vi "test_Add Command_Check Existing Command Parameters Are Overwritten.vi"(8 "error in (no error)":errorcluster, 11 "TestCase in":refnum<class "Instrument Addon Scripting API Messages Unit Tests.lvclass">) -> (0 "error out":errorcluster, 3 "TestCase out":refnum<class "Instrument Addon Scripting API Messages Unit Tests.lvclass">)   [LabVIEW 2018, in "Instrument Addon Scripting API Messages Unit Tests.lvclass"]
uses:
  Instrument Addon Scripting API Messages Unit Tests.lvclass
  APIs/Scripting API/TypeDefs/Command Settings.ctl
  <vilib>/NI Veristand/Custom Device API/Custom Device Item Ref.ctl
  APIs/Scripting API/TypeDefs/Padding.ctl
  Addon/Addon Shared/Types/FG Control.ctl
  Addon/Addon Shared/Types/Command Parameters.ctl
  Addon/Addon Shared/Types/Linked Channel Cluster.ctl
  Instrument Addon Scripting API Messages Unit Tests.lvclass/Instrument Addon Scripting API Messages Unit Tests.ctl
  Addon/Addon Shared/SubVIs/Constants.vi
  <vilib>/NI/NI VeriStand Advanced SysDef API/_SubVIs/SysDef.Search.GUID.vi
  <vilib>/NI Veristand/Custom Device API/NI VeriStand - Get Item Property.vi
  <vilib>/NI Veristand/Custom Device API/Get Item Property (String).vi
  <vilib>/NI Veristand/Custom Device API/Get Item Property (String Array).vi
  <vilib>/NI Veristand/Custom Device API/Get Item Property (Boolean).vi
  <vilib>/NI Veristand/Custom Device API/Get Item Property (U32).vi
  <vilib>/NI Veristand/Custom Device API/NI VeriStand - Set Item Property.vi
  <vilib>/NI Veristand/Custom Device API/Set Item Property (String).vi
  <vilib>/NI Veristand/Custom Device API/Set Item Property (String Array).vi
  <vilib>/NI Veristand/Custom Device API/Set Item Property (Boolean).vi
  <vilib>/NI Veristand/Custom Device API/Set Item Property (U32).vi
  <vilib>/addons/_JKI Toolkits/VI Tester/TestCase.llb/TestCase.lvclass
  Instrument Addon Scripting API Test Assets/Instrument Addon Scripting API Test Assets.lvclass
  Addon/Addon Shared/Instrument Addon Shared.lvlib
  <vilib>/NI/NI VeriStand Advanced SysDef API/SysDef API/Advanced System Definition.lvlib
  <vilib>/NI Veristand/Custom Device API/Custom Device API.lvlib
  APIs/Scripting API/Instrument Addon Scripting API.lvlib
  C:/Program Files (x86)/National Instruments/LabVIEW 2018/vi.lib/addons/_JKI Toolkits/VI Tester/TestCase.llb/TestCase.lvclass
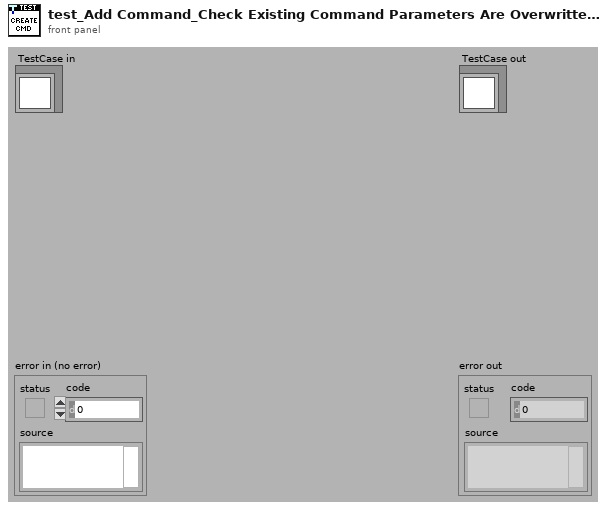
[diagram p1: front panel]
types:
  T1 = typedef "Instrument Addon Shared.lvlib/FG Control.ctl" = enum16{"Get", "Set"}
  T2 = typedef "Instrument Addon Scripting API.lvlib/Command Settings.ctl" = cluster{"Command Format":string, "Linked Channels":cluster{"Variable Name":string, "Channel Ref in":T3}[], "Use Padding?":bool, "Padding":T4}
  T3 = typedef "Custom Device API.lvlib/Custom Device Item Ref.ctl" = u64
  T4 = typedef "Instrument Addon Scripting API.lvlib/Padding.ctl" = cluster{"Pad Value":u8, "Length":u32}
  T5 = typedef "Instrument Addon Shared.lvlib/Command Parameters.ctl" = cluster{"Command":string, "Linked Channels":T6[], "Pad":bool, "Length":u32, "Pad Value":u8}
  T6 = typedef "Instrument Addon Shared.lvlib/Linked Channel Cluster.ctl" = cluster{"Variable Name":string, "GUID":string}
  T7 = typedef "Instrument Addon Scripting API.lvlib/Linked Channel.ctl" = cluster{"Variable Name":string, "Channel Refnum":T3}
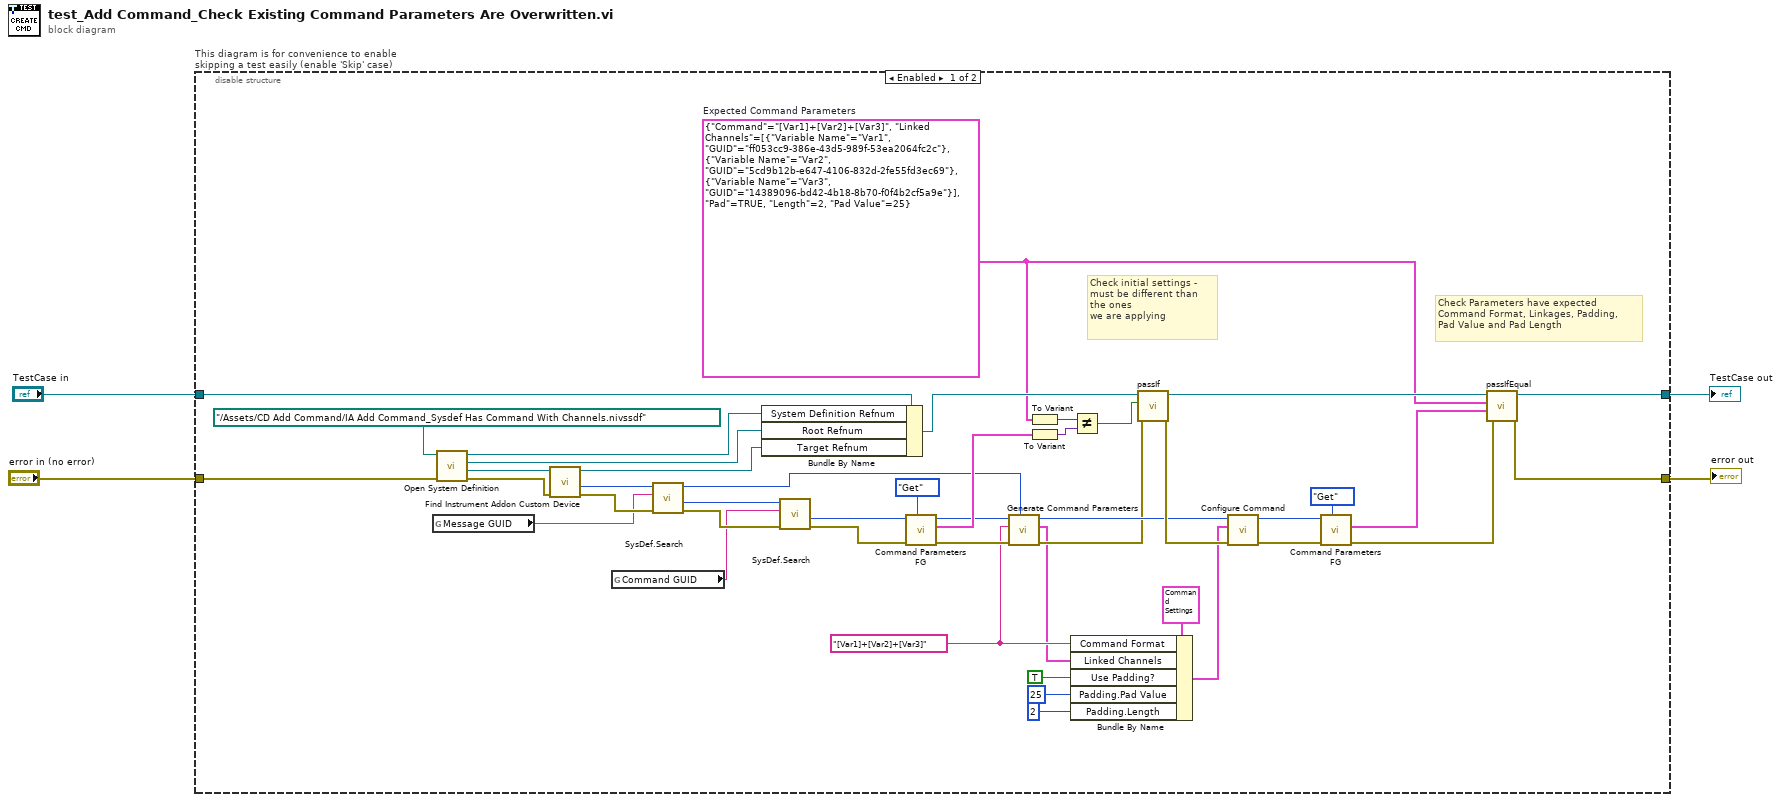
[diagram p0: block diagram]
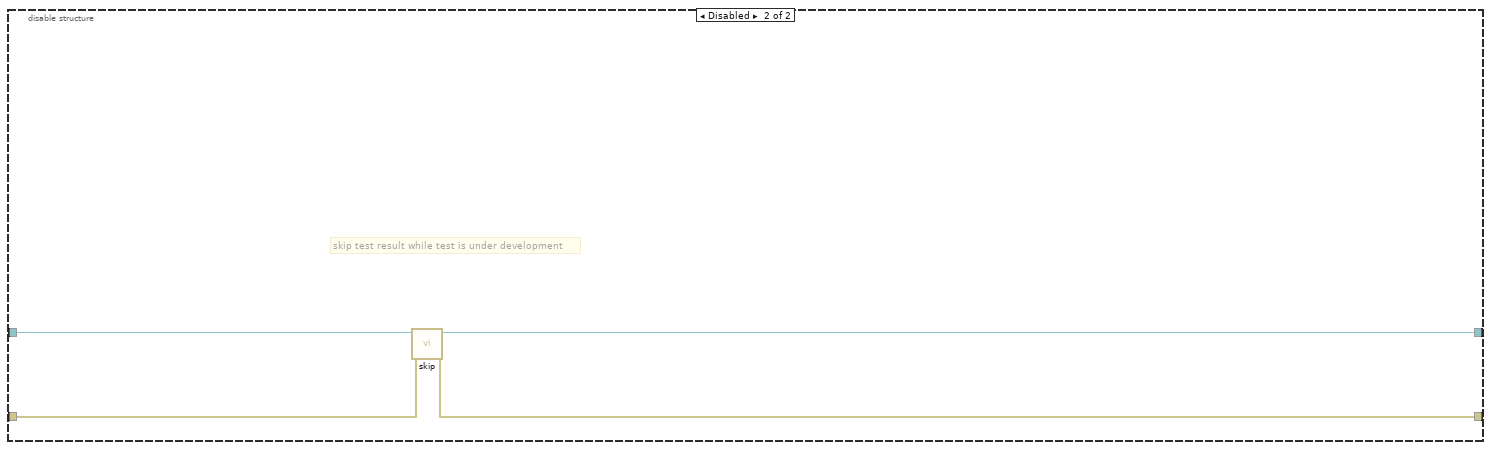
[diagram p2: hidden frame]
diagram:
  n1 = disable-structure "This diagram is for convenience to enable skipping a test easily (enable 'Skip' case)" shown="Enabled" {
    disable-tunnel: "TestCase in" -> [w21 w52]
    disable-tunnel: [w45 w50] -> w1
    disable-tunnel: [w46 w51] -> w3
    disable-tunnel: "error in (no error)" -> [w47 w49]
    frame Enabled {
      w5 = T5 {"Command"="[Var1]+[Var2]+[Var3]", "Linked Channels"=[{"Variable Name"="Var1", "GUID"="ff053cc9-386e-43d5-989f-53ea2064fc2c"}, {"Variable Name"="Var2", "GUID"="5cd9b12b-e647-4106-832d-2fe55fd3ec69"}, {"Variable Name"="Var3", "GUID"="14389096-bd42-4b18-8b70-f0f4b2cf5a9e"}], "Pad"=TRUE, "Length"=2, "Pad Value"=25}  # Expected Command Parameters
      w7 = "[Var1]+[Var2]+[Var3]" ("Command Format")
      # "Check initial settings - must be different than the ones\nwe are applying"
      # "Check Parameters have expected \nCommand Format, Linkages, Padding,\nPad Value and Pad Length"
      n2 = global read "Constants.vi" "Message GUID"() -> (w38:string)
      n3 = call "Open System Definition.vi"("error in (no error)"=w47, "System Definition File"=path "../Assets/CD Add Command/IA Add Command_Sysdef Has Command With Channels.nivssdf" ("SDF file")) -> ("error out"=w40:errorcluster, "Target Refnum"=w41:refnum<k24>, "Root Refnum"=w18:refnum<k24>, "System Definition Refnum"=w19:refnum<k24>)  [unwired: 6 in]
      n4 = call "Find Instrument Addon Custom Device.vi"("error in"=w40, "target in"=w41) -> ("error out"=w39:errorcluster, "NodeID"=w36:u64, "target out"=w17:refnum<k24>)  [unwired: 7 in]
      n5 = global read "Constants.vi" "Command GUID"() -> (w33:string)
      n6 = call-poly <vilib>:"SysDef.Search.vi"("error in (no error)"=w39, "GUID"=w38, "nodeID"=w36) -> ("error out"=w35:errorcluster, "Value out"=w34:u64, "nodeID out"=w8:u64)  [unwired: 5 in, 1 out]
      n7 = Bundle By Name(cluster=w21, "System Definition Refnum"=w19, "Root Refnum"=w18, "Target Refnum"=w17) -> (w20:refnum<class "Instrument Addon Scripting API Messages Unit Tests.lvclass">)
      n8 = call-poly <vilib>:"SysDef.Search.vi"("error in (no error)"=w35, "GUID"=w33, "nodeID"=w34) -> ("error out"=w31:errorcluster, "Value out"=w32:u64)  [unwired: 5 in, 2 out]
      n9 = call "Command Parameters FG.vi"("Action"=FG_Control."Get", "error in (no error)"=w31, "Item Ref in"=w32) -> ("error out"=w10:errorcluster, "Command Parameters"=w25:T5, "Item Ref out"=w12:T3)  [unwired: 6 in]
      n10 = call "Generate Command Parameters.vi"("Instrument Addon Refnum in"=w8, "Error In"=w10, "Command String"=w7, "Command Channel in"=w12) -> ("Error Out"=w9:errorcluster, "Linked Channels"=w6:T7[], "Command Channel out"=w11:T3)  [unwired: 4 in, 1 out]
      n11 = To Variant(anything=w5) -> (Variant=w28:variant)
      n12 = To Variant(anything=w25) -> (Variant=w27:variant)
      n13 = Bundle By Name(cluster=T2 {"Command Format"="[Var1]+[Var2]", "Linked Channels"=[{"Variable Name"="Var1", "Channel Ref in"=32}, {"Variable Name"="Var2", "Channel Ref in"=33}], "Use Padding?"=FALSE, "Padding"={"Pad Value"=0, "Length"=0}} ("Settings"), "Command Format"=w7, "Linked Channels"=w6, "Use Padding?"=TRUE, "Padding.Pad Value"=u8 25, "Padding.Length"=u32 2) -> (w14:T2)
      n14 = Not Equal?(x=w28, y=w27) -> (x != y?=w26:bool)
      n15 = call-dynamic "passIf.vi"("error in (no error)"=w9, "pass"=w26, "TestCase in"=w20) -> ("error out"=w16:errorcluster, "TestCase out"=w29:refnum<class "Instrument Addon Scripting API Messages Unit Tests.lvclass">)  [unwired: 7 in]
      n16 = call "Configure Command.vi"("error in (no error)"=w16, "settings"=w14, "command refnum in"=w11) -> ("error out"=w15:errorcluster, "command refnum out"=w13:T3)  [unwired: 7 in]
      n17 = call "Command Parameters FG.vi"("Action"=FG_Control."Get", "error in (no error)"=w15, "Item Ref in"=w13) -> ("error out"=w43:errorcluster, "Command Parameters"=w42:T5)  [unwired: 6 in, 1 out]
      n18 = call-dynamic "passIfEqual.vi"("error in (no error)"=w43, "y"=w42, "x"=w5, "TestCase in"=w29) -> ("error out"=w46:errorcluster, "TestCase out"=w45:refnum<class "Instrument Addon Scripting API Messages Unit Tests.lvclass">)  [unwired: 6 in]
    }
    frame Disabled {
      # "skip test result while test is under development"
      n19 = call <vilib>:"skip.vi"("error in (no error)"=w49, "TestCase in"=w52) -> ("error out"=w51:errorcluster, "TestCase out"=w50:refnum<class "Instrument Addon Scripting API Messages Unit Tests.lvclass">)  [unwired: 8 in]
    }
  }
  "error out" <- w3
  "TestCase out" <- w1
